vi "Error cluster to error response.vi"(7 "status in":string="OK", 8 "error in (no error)":errorcluster, 11 "response":string) -> (2 "JSON String":string, 3 "message":string)   [LabVIEW 2019]
doc: "Converts standard LV error cluster to error response JSON string"
uses:
  <vilib>/Utility/error.llb/DialogType.ctl
  Error response.ctl
  CommandResponse communication.lvlib
  <vilib>/addons/_JKI.lib/Serialization/JSON/JKI JSON Serialization.lvlib
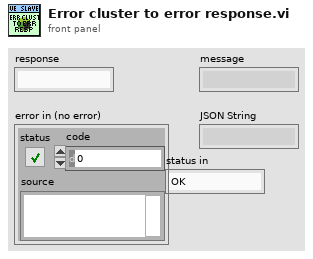
[diagram p1: front panel]
types:
  T1 = typedef "CommandResponse communication.lvlib/Error response.ctl" = cluster{"code":i32, "message":string, "source":string}
  T2 = typedef "DialogType.ctl" = u16
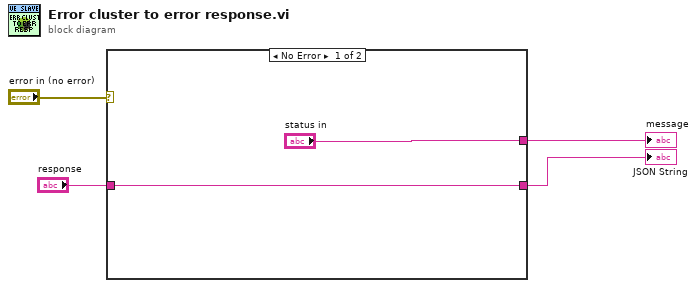
[diagram p0: block diagram]
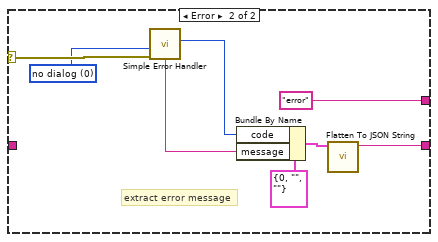
[diagram p2: hidden frame]
diagram:
  n1 = case shown="No Error" "error in (no error)" {
    selector: "error in (no error)" -> [_ w13]
    tunnel: ["status in" "error" ("message")] -> w1
    tunnel: [w5 w7] -> w3
    tunnel: "response" -> [w5 _]
    frame No Error {
    }
    frame Error {
      w12 = T2 0 items=["no dialog", "OK message", "continue or stop message", "OK message + warnings", "continue/stop + warnings"] ("type of dialog (OK msg:1)")
      # "extract error message"
      n2 = call <vilib>:"Simple Error Handler.vi"("type of dialog (OK msg:1)"=w12, "error in (no error)"=w13) -> ("code out"=w10:i32, "message"=w9:string)  [unwired: 3 in, 3 out]
      n3 = Bundle By Name(cluster=T1 {"code"=0, "message"="", "source"=""} ("Error response"), "code"=w10, "message"=w9) -> (w8:T1)
      n4 = call <vilib>:"Flatten To JSON String.vi"("Variant"=w8) -> ("JSON String"=w7:string)  [unwired: 9 in, 1 out]
    }
  }
  "JSON String" <- w3
  "message" <- w1
